vi "Async.Engine.Write Data to HW.vi"(8 "error in (no error)":errorcluster, 11 "VS Inline Async API in":refnum<class "VS Inline Async API.lvclass">) -> (0 "error out":errorcluster, 3 "VS Inline Async API out":refnum<class "VS Inline Async API.lvclass">)   [LabVIEW 2023, in "VS Inline Async API.lvlib" / "VS Inline Async API.lvclass"]
uses:
  VS Inline Async API.lvclass
  VS Inline Async API.lvclass/VS Inline Async API.ctl
  _Data Access Engine/Data Access Engine/Data Access Engine.lvclass/Data Access Engine.ctl
  _Data Access Engine/Access Type Classes/Read/Read.lvclass/Read.ctl
  _Data Access Engine/Data Access Engine/Data Access Engine.lvclass
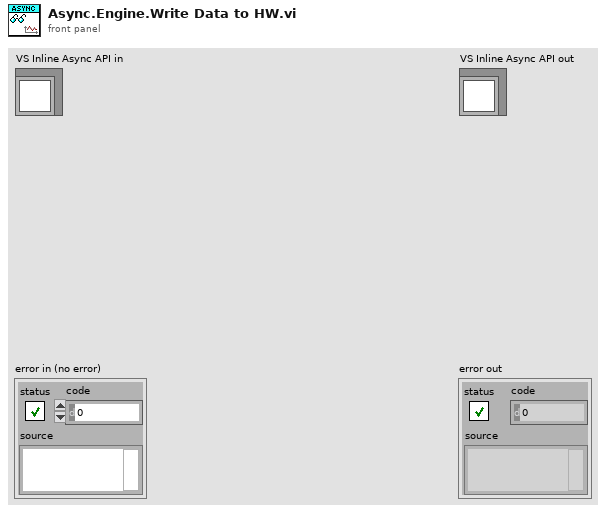
[diagram p1: front panel]
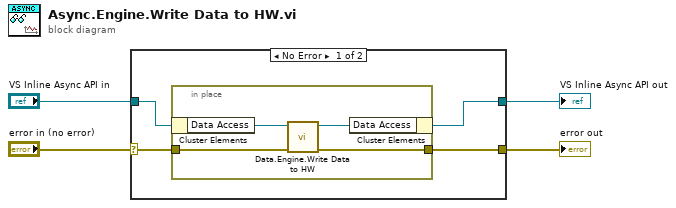
[diagram p0: block diagram]
diagram:
  n1 = case shown="No Error" "error in (no error)" {
    selector: "error in (no error)" -> [w6 w14]
    tunnel: [w5 w14] -> w3
    tunnel: [w7 w13] -> w1
    tunnel: "VS Inline Async API in" -> [w8 w13]
    frame No Error {
      n2 = in-place {
        in-place-border: w6 -> [w12]
        in-place-border: [w9] -> w5
        n3 = in-place-cluster #1(w8) -> ("Data Access"=w11:refnum<class "Data Access Engine.lvclass">)
        n4 = call "Data.Engine.Write Data to HW.vi"("error in (no error)"=w12, "Data Access API in"=w11) -> ("error out"=w9:errorcluster, "Data Access API out"=w10:refnum<class "Data Access Engine.lvclass">)  [unwired: 8 in]
        n5 = in-place-cluster #1("Data Access"=w10) -> (w7:refnum<class "VS Inline Async API.lvclass">)
      }
    }
    frame Error {
    }
  }
  "error out" <- w3
  "VS Inline Async API out" <- w1
